vi "Transition.vi"(6 "Kind":enum16{"External", "Local", "Internal"}(ring)=enum."Internal", 8 "error in (no error)":errorcluster, 9 "Target State":refnum<class "State.lvclass">, 10 "Context in":refnum<data-value>, 11 "State in":refnum<class "State.lvclass">) -> (0 "error out":errorcluster, 2 "Context out":refnum<data-value>, 3 "State out":refnum<class "State.lvclass">)   [LabVIEW 2024, in "State.lvlib" / "State.lvclass"]
uses:
  State.lvclass
  Context/Context/Context.lvclass
  Nested State/Nested State.lvclass
  C:/Users/uspoaotto/OneDrive - Oregon Tool/Desktop/temp/actor framework state machine/State Machine/State/State/State.lvclass
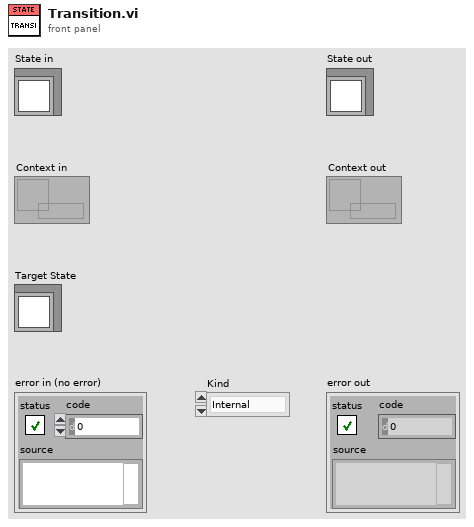
[diagram p1: front panel]
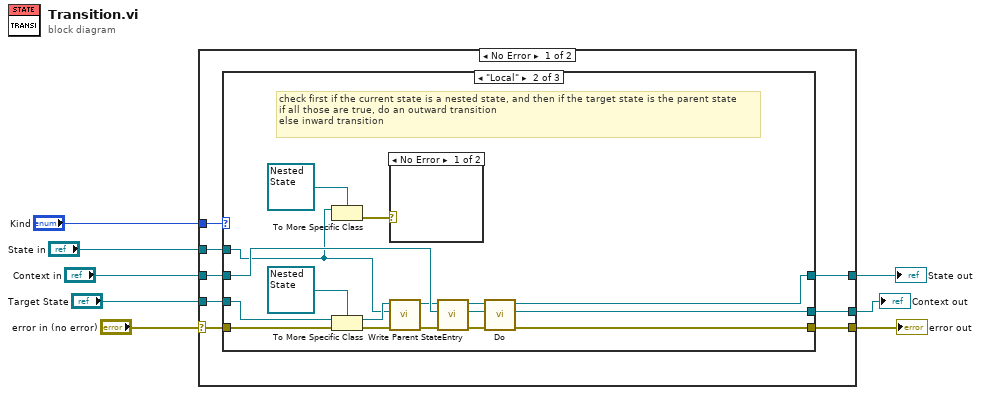
[diagram p0: block diagram]
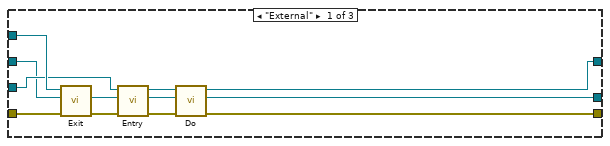
[diagram p2: hidden frame]
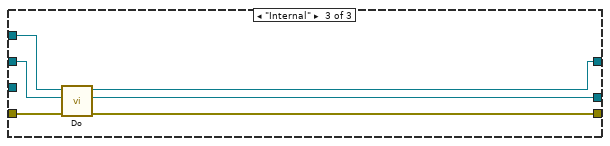
[diagram p4: hidden frame]
diagram:
  n1 = case shown="No Error" "error in (no error)" {
    selector: "error in (no error)" -> [w13 w54]
    tunnel: [w12 w54] -> w7
    tunnel: [w16 w53] -> w5
    tunnel: "State in" -> [w15 w53]
    tunnel: "Kind" -> [w11 _]
    tunnel: "Target State" -> [w14 _]
    tunnel: "Context in" -> [w10 w52]
    tunnel: [w9 w52] -> w1
    frame No Error {
      n2 = case shown="\"Local\"" w11 {
        tunnel: [w27 w43 w48] -> w16
        tunnel: w15 -> [w26 w29 w51]
        tunnel: w14 -> [w21 w36 _]
        tunnel: w13 -> [w24 w34 w50]
        tunnel: [w22 w44 w49] -> w12
        tunnel: w10 -> [w20 w41 w47]
        tunnel: [w17 w39 w46] -> w9
        frame "External" {
          n3 = call-dynamic "Exit.vi"("error in (no error)"=w24, "Context in"=w20, "State in"=w26) -> ("error out"=w25:errorcluster, "Context out"=w19:refnum<data-value>)  [unwired: 6 in, 1 out]
          n4 = call-dynamic "Entry.vi"("error in (no error)"=w25, "Context in"=w19, "State in"=w21) -> ("error out"=w23:errorcluster, "Context out"=w18:refnum<data-value>, "State out"=w28:refnum<class "State.lvclass">)  [unwired: 6 in]
          n5 = call-dynamic "Do.vi"("error in (no error)"=w23, "Context in"=w18, "State in"=w28) -> ("error out"=w22:errorcluster, "Context out"=w17:refnum<data-value>, "State out"=w27:refnum<class "State.lvclass">)  [unwired: 6 in]
        }
        frame "Local" {
          # "check first if the current state is a nested state, and then if the target state is the parent state\nif all those are true, do an outward transition\nelse inward transition"
          n6 = To More Specific Class(target class=refnum<class "Nested State.lvclass"> refnum ("State.lvlib:Nested State.lvclass"), reference=w29) -> (error out=w30:errorcluster)  [unwired: 1 in, 1 out]
          n7 = To More Specific Class(target class=refnum<class "Nested State.lvclass"> refnum ("State.lvlib:Nested State.lvclass"), reference=w36, error in=w34) -> (specific class reference=w35:refnum<class "Nested State.lvclass">, error out=w38:errorcluster)
          n8 = case shown="No Error" w30 {
            frame No Error {
            }
            frame Error {
            }
          }
          n9 = call-dynamic "Write Parent State.vi"("error in (no error)"=w38, "Parent State"=w29, "Nested State in"=w35) -> ("error out"=w32:errorcluster, "Nested State out"=w33:refnum<class "Nested State.lvclass">)  [unwired: 7 in]
          n10 = call-dynamic "Entry.vi"("error in (no error)"=w32, "Context in"=w41, "State in"=w33) -> ("error out"=w45:errorcluster, "Context out"=w40:refnum<data-value>, "State out"=w42:refnum<class "Nested State.lvclass">)  [unwired: 6 in]
          n11 = call-dynamic "Do.vi"("error in (no error)"=w45, "Context in"=w40, "State in"=w42) -> ("error out"=w44:errorcluster, "Context out"=w39:refnum<data-value>, "State out"=w43:refnum<class "Nested State.lvclass">)  [unwired: 6 in]
        }
        frame "Internal" {
          n12 = call-dynamic "Do.vi"("error in (no error)"=w50, "Context in"=w47, "State in"=w51) -> ("error out"=w49:errorcluster, "Context out"=w46:refnum<data-value>, "State out"=w48:refnum<class "State.lvclass">)  [unwired: 6 in]
        }
      }
    }
    frame Error {
    }
  }
  "error out" <- w7
  "State out" <- w5
  "Context out" <- w1
